vi "DaNIDemoVIveryveryfinal.vi"() -> ()   [LabVIEW 2016]
uses:
  <vilib>/userdefined/High Color/nirio_resource_hc.ctl
  <vilib>/imath/engines/lvmath2/RunTimeEngine/Managers/WorkSpace/UID Generator.vi
  <vilib>/imath/engines/lvmath2/RunTimeEngine/RunTimeType/NIMS_RunTimeType_From StrictType (excl LVString).vi
  <instcachedir>/0/NIMS_RunTimeType_From StrictType (excl LVString)_BBF44FB49F834B71AF7A14CCEDF8BECD.lvgen/NIMS_RunTimeType_From StrictType (excl LVString)_BBF44FB49F834B71AF7A14CCEDF8BECD_000.vi
  <vilib>/imath/engines/lvmath2/RunTimeEngine/LocalVariableDefStatement/MC_LocalVariableDefStatement_Display.vi
  <vilib>/imath/engines/lvmath2/RunTimeEngine/Managers/SymbolTable/Clear UID.vi
  <vilib>/imath/engines/lvmath2/RunTimeEngine/NodeEndStatement/NIMS_NodeEndStatement_Output.vi
  <instcachedir>/0/NIMS_NodeEndStatement_Output_53EC0D466D134D7ABD903AC30B43404B.lvgen/NIMS_NodeEndStatement_Output_53EC0D466D134D7ABD903AC30B43404B_001.vi
  <vilib>/imath/engines/lvmath2/RunTimeEngine/ErrorHandling/NIMS_Finalize Error.vi
  <vilib>/imath/engines/lvmath2/RunTimeEngine/Managers/SymbolTable/NIMS_WorkSpace.lvlib
panel:
  out "x .or. y?":bool
  out "wddot":dbl
  out "vddot":dbl
  in  "Stop Button":bool
  in  "Mode Select":T1(ring)=enum."DaNI Simulation"
  in  "IP Adress":T2="rio://169.254.0.1/RIO0"
  in  "dt (ms)":u32=65
  out "Rad/s Left":dbl
  out "Rad/s Right":dbl
  in  "Left _PID":cluster{"Kp":dbl, "Ti":dbl, "Td":dbl}={"Kp"=0.035, "Ti"=1.25, "Td"=0.0001}
  in  "Right_PID":cluster{"Kp":dbl, "Ti":dbl, "Td":dbl}={"Kp"=0.035, "Ti"=1.5, "Td"=0.0001}
  out "s1 and s2":cluster{"ve":dbl, "we":dbl}(graph)
  out "thetad":dbl
  out "yd":dbl
  out "xd":dbl
  out "w_L":dbl
  out "w_R":dbl
  out "wd":dbl
  out "vd":dbl
  in  "k":cluster{" k0":dbl, "k1":dbl, "k2":dbl}={" k0"=2.0, "k1"=4.0, "k2"=1.1}
  in  "file path (use dialog)":path
  out "error in v and w":cluster{"ve":dbl, "we":dbl}(graph)
  out "error in x y theta":cluster{"xe":dbl, "ye":dbl, "thetae":dbl}(graph)
  out "desired and controlled w":cluster{dbl, "xr+1":dbl}(graph)
  out "desired and controlled v":cluster{dbl, "xr+1":dbl}(graph)
  out "desired and controlled theta":cluster{dbl, "xr+1":dbl}(graph)
  out "desired and controlled trajectory":cluster{dbl[], dbl[]}[](graph)
  out "desired y and controlled y":cluster{dbl, "yr+1":dbl}(graph)
  out "desired x and controlled x":cluster{dbl, "xr+1":dbl}(graph)
  in  "P and Q":cluster{"P1":dbl, "P2":dbl, "Q1":dbl, "Q2":dbl}={"P1"=0.2, "P2"=0.2, "Q1"=0.4, "Q2"=0.4}
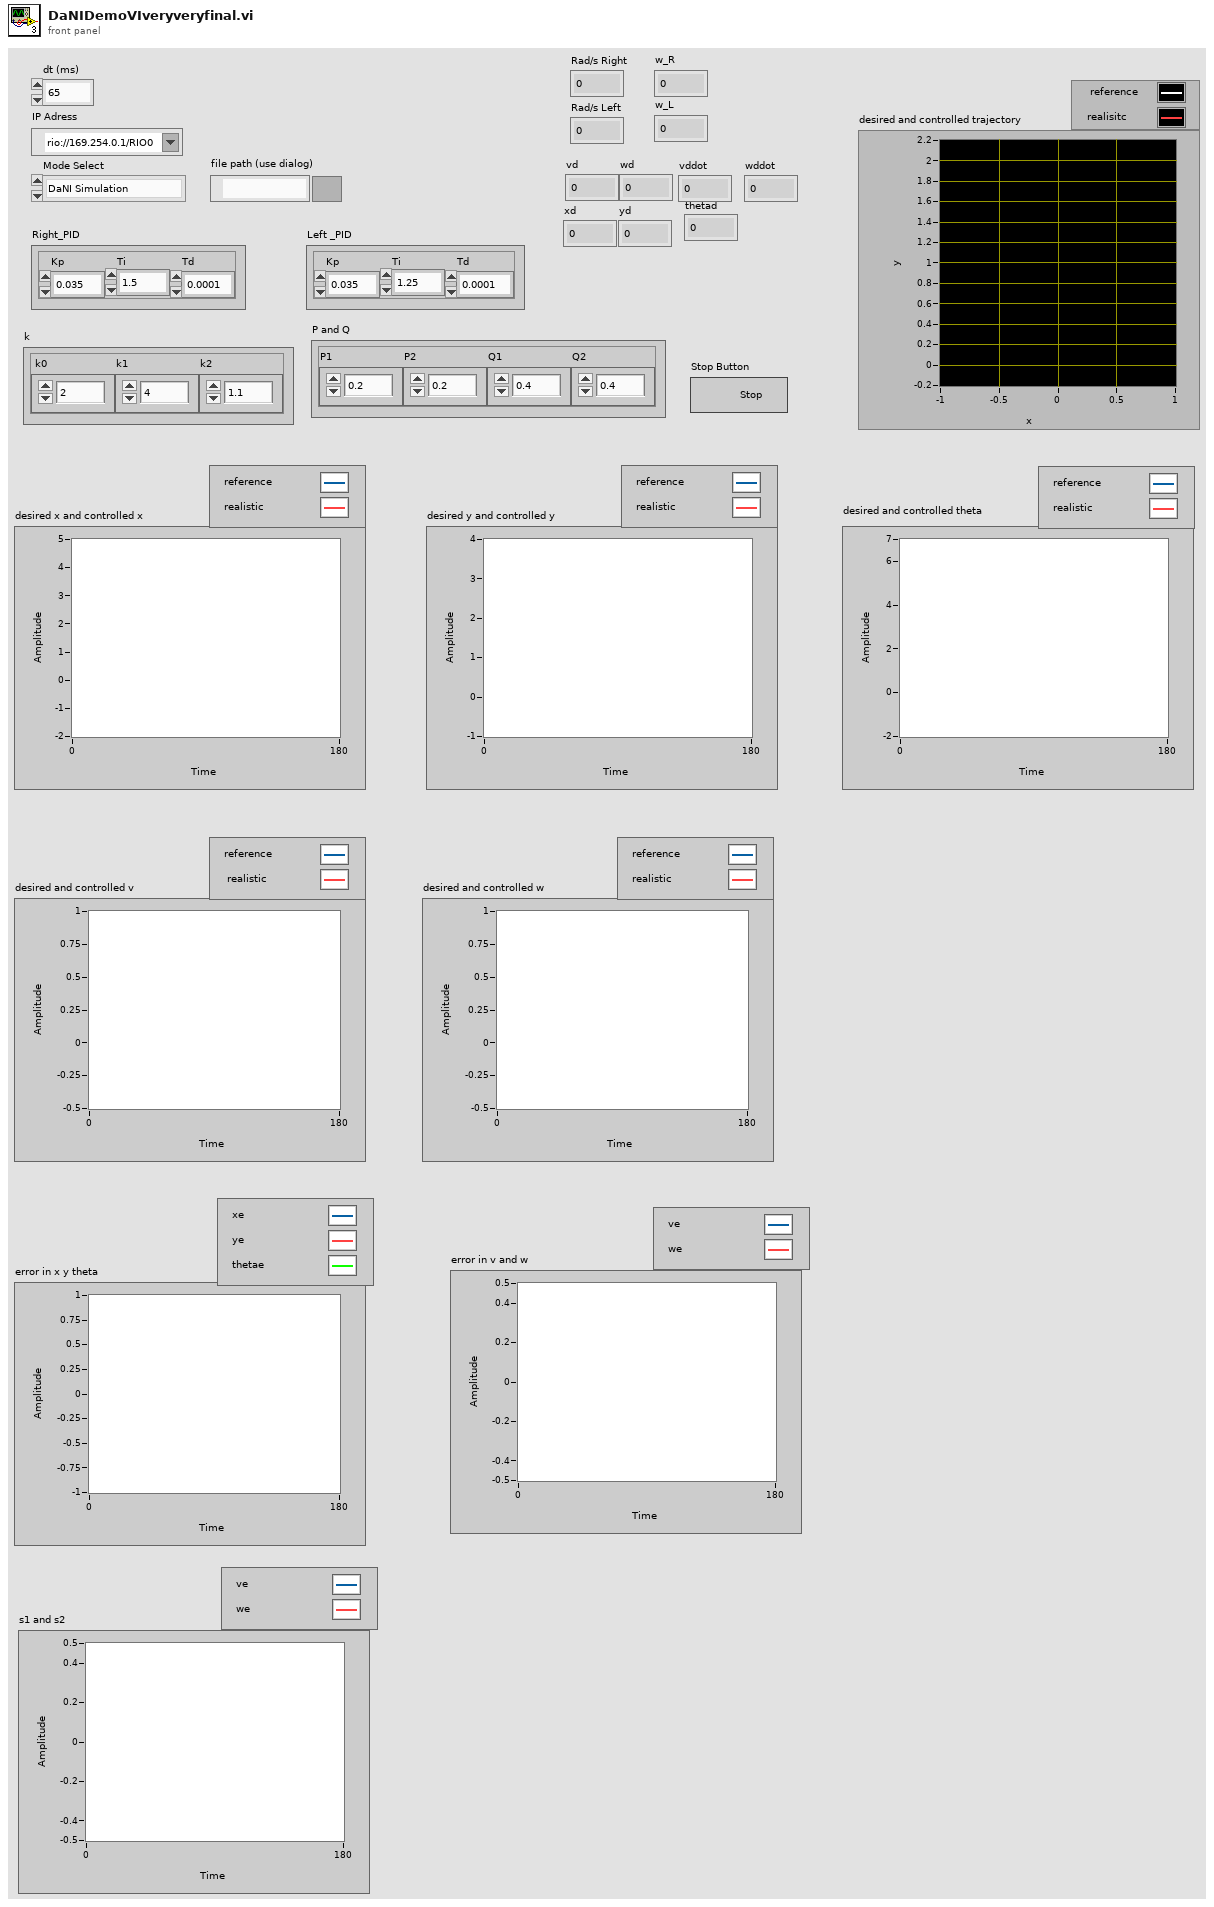
[diagram p1: front panel]
types:
  T1 = enum16{"DaNI DC Motor Sim", "DaNI Simulation", "DaNI Robot"}
  T2 = typedef "nirio_resource_hc.ctl" = tag
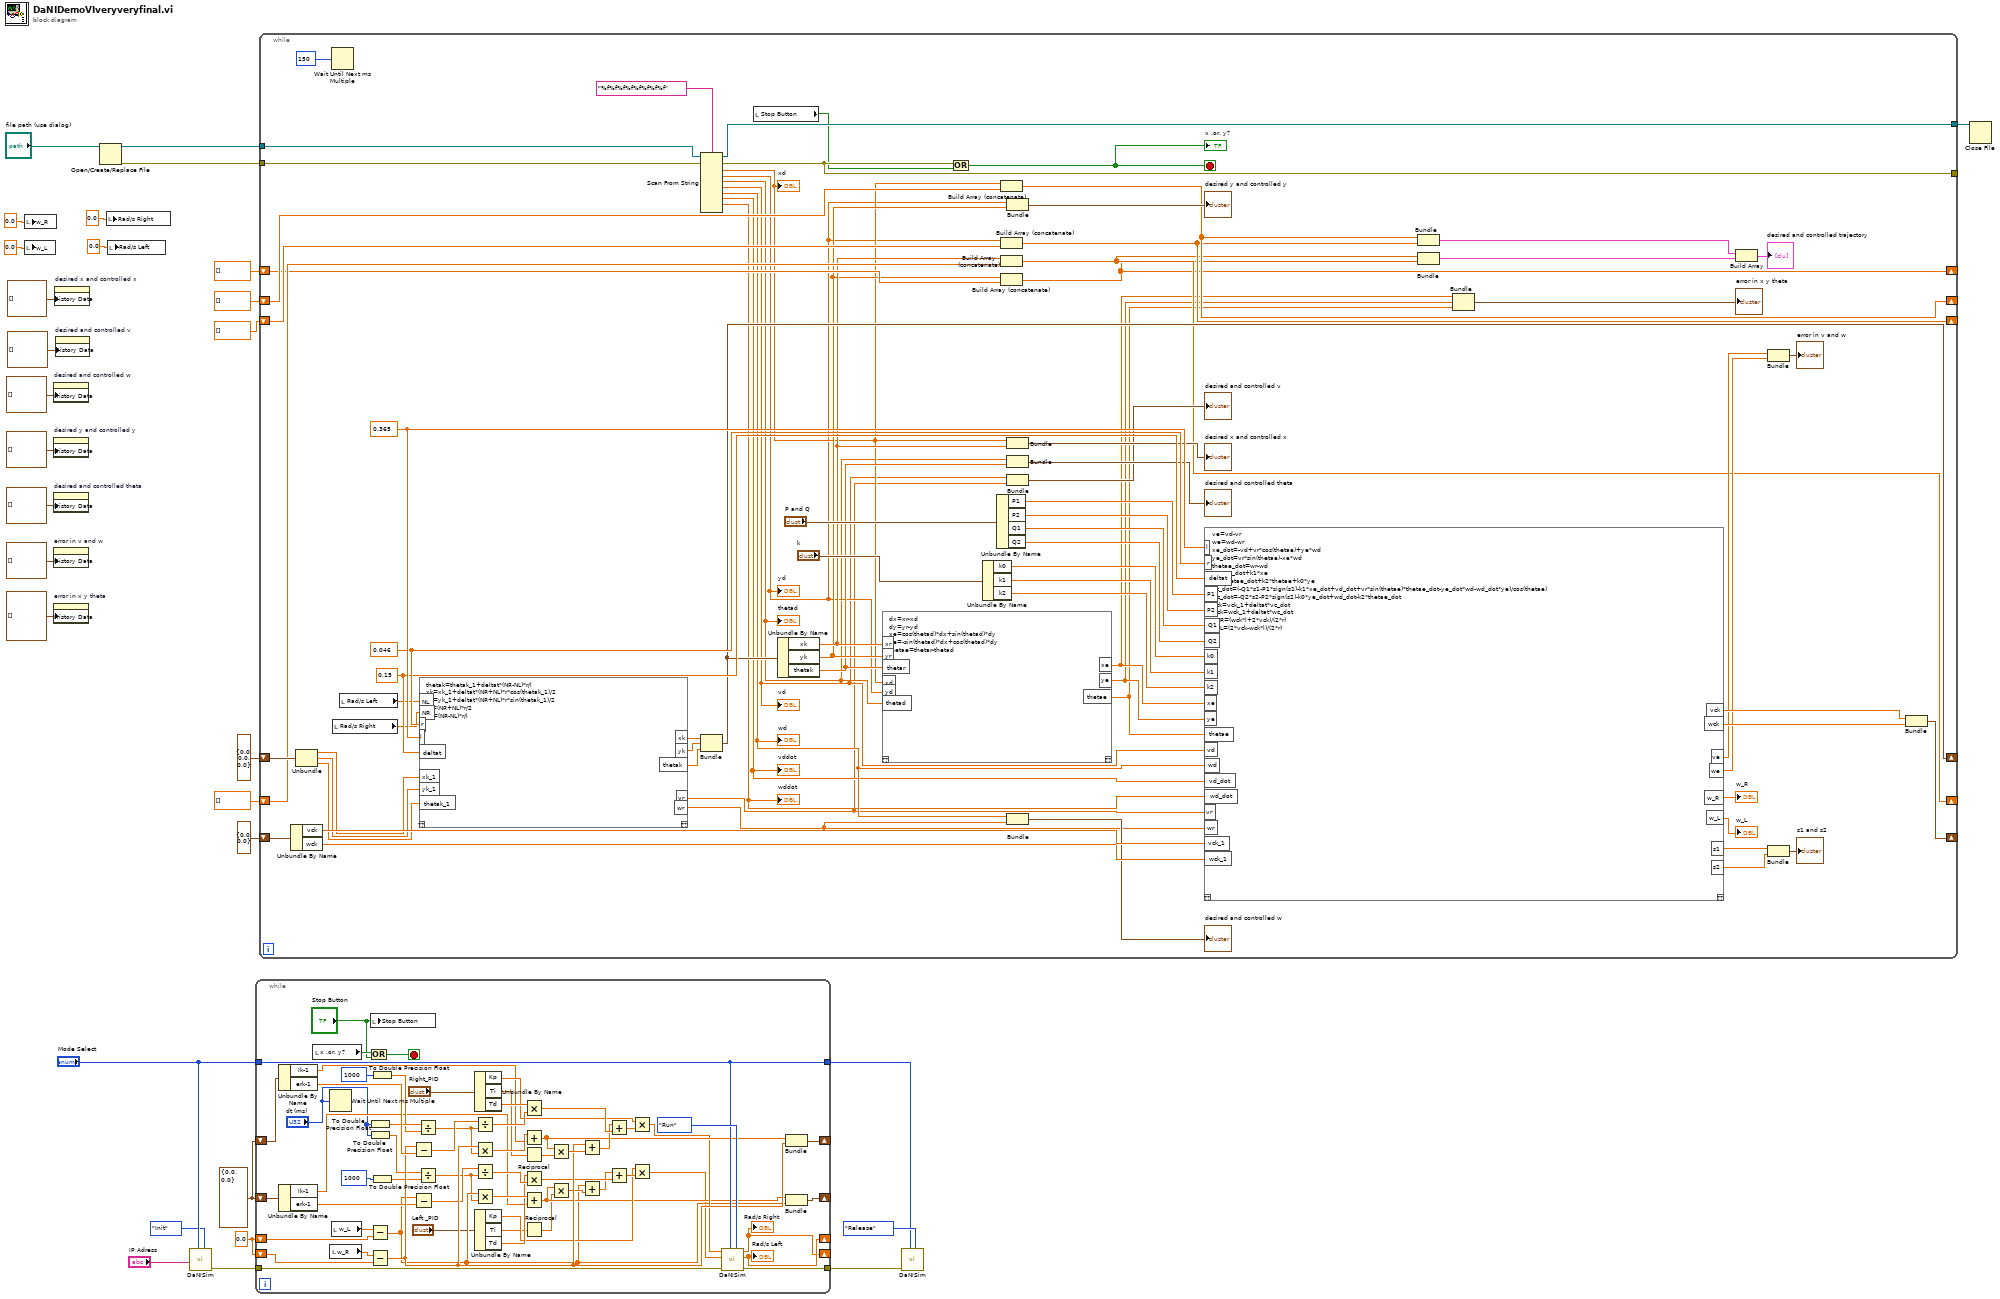
[diagram p0: block diagram]
diagram:
  w9 = 0.0 ("OmegaR")
  w13 = cluster{"Ik-1":dbl, "erk-1":dbl} {"Ik-1"=0.0, "erk-1"=0.0} ("tk-1")
  n1 = local write "w_R"(0.0 ("w_R")) -> ()
  n2 = local write "w_L"(0.0 ("w_L")) -> ()
  n3 = property on="desired and controlled w" class="WFChart (strict)"("History Data"=cluster{dbl, "xr+1":dbl}[] []) -> ()  [unwired: 2 in, 2 out]
  n4 = property on="desired y and controlled y" class="WFChart (strict)"("History Data"=cluster{dbl, "yr+1":dbl}[] []) -> ()  [unwired: 2 in, 2 out]
  n5 = property on="desired and controlled theta" class="WFChart (strict)"("History Data"=cluster{dbl, "xr+1":dbl}[] []) -> ()  [unwired: 2 in, 2 out]
  n6 = property on="error in v and w" class="WFChart (strict)"("History Data"=cluster{"ve":dbl, "we":dbl}[] []) -> ()  [unwired: 2 in, 2 out]
  n7 = property on="error in x y theta" class="WFChart (strict)"("History Data"=cluster{"xe":dbl, "ye":dbl, "thetae":dbl}[] []) -> ()  [unwired: 2 in, 2 out]
  n8 = property on="desired x and controlled x" class="WFChart (strict)"("History Data"=cluster{dbl, "xr+1":dbl}[] []) -> ()  [unwired: 2 in, 2 out]
  n9 = property on="desired and controlled v" class="WFChart (strict)"("History Data"=cluster{dbl, "xr+1":dbl}[] []) -> ()  [unwired: 2 in, 2 out]
  n10 = Open/Create/Replace File(file path (use dialog)="file path (use dialog)") -> (refnum out=w29:refnum<file>, error out=w28:errorcluster)  [unwired: 5 in, 1 out]
  n11 = local write "Rad/s Right"(0.0 ("Rad/s Left")) -> ()
  n12 = local write "Rad/s Left"(0.0 ("Rad/s Right")) -> ()
  n13 = call "DaNISim.vi"("Action"=enum16{"Init", "Run", "Release"}."Init", "Mode Select"="Mode Select", "IP Adress"="IP Adress") -> ("error out"=w5:errorcluster)  [unwired: 5 in, 3 out]
  n14 = while {
    tunnel: w5 -> [w90]
    tunnel: "Mode Select" -> [w85]
    tunnel: [w89] -> w11
    tunnel: [w85] -> w10
    shift-right: [w41] -> _
    shift-left: w13 -> [w40]
    shift-right: [w61] -> _
    shift-left: w13 -> [w62]
    shift-right: [w87] -> _
    shift-left: w9 -> [w65]
    shift-right: [w88] -> _
    shift-left: w9 -> [w37]
    stop <- w31 stop-if-true
    n15 = Unbundle By Name(w62) -> ("Ik-1"=w75:dbl, "erk-1"=w74:dbl)
    n16 = Unbundle By Name(w40) -> ("Ik-1"=w50:dbl, "erk-1"=w49:dbl)
    n17 = local read "x .or. y?"() -> (w33:bool)
    n18 = Wait Until Next ms Multiple(millisecond multiple="dt (ms)") -> ()  [unwired: 1 out]
    n19 = local read "w_R"() -> (w64:dbl)
    n20 = local read "w_L"() -> (w38:dbl)
    n21 = Or(x=w33, y="Stop Button") -> (x .or. y?=w31:bool)
    n22 = To Double Precision Float(number="dt (ms)") -> (double precision float=w70:dbl)
    n23 = To Double Precision Float(number="dt (ms)") -> (double precision float=w45:dbl)
    n24 = Subtract(x=w38, y=w37) -> (x-y=w47:dbl)
    n25 = Subtract(x=w64, y=w65) -> (x-y=w72:dbl)
    n26 = local write "Stop Button"("Stop Button") -> ()
    n27 = To Double Precision Float(number=1000) -> (double precision float=w69:dbl)
    n28 = To Double Precision Float(number=1000) -> (double precision float=w44:dbl)
    n29 = Subtract(x=w72, y=w74) -> (x-y=w83:dbl)
    n30 = Subtract(x=w47, y=w49) -> (x-y=w58:dbl)
    n31 = Divide(x=w70, y=w69) -> (x/y=w66:dbl)
    n32 = Divide(x=w45, y=w44) -> (x/y=w43:dbl)
    n33 = Unbundle By Name("Right_PID") -> ("Kp"=w76:dbl, "Ti"=w68:dbl, "Td"=w77:dbl)
    n34 = Divide(x=w83, y=w66) -> (x/y=w84:dbl)
    n35 = Multiply(x=w72, y=w66) -> (x*y=w79:dbl)
    n36 = Divide(x=w58, y=w43) -> (x/y=w59:dbl)
    n37 = Multiply(x=w47, y=w43) -> (x*y=w54:dbl)
    n38 = Unbundle By Name("Left _PID") -> ("Kp"=w51:dbl, "Ti"=w35:dbl, "Td"=w52:dbl)
    n39 = Multiply(x=w77, y=w84) -> (x*y=w82:dbl)
    n40 = Add(x=w79, y=w75) -> (x+y=w73:dbl)
    n41 = Reciprocal(x=w68) -> (1/x=w67:dbl)
    n42 = Multiply(x=w52, y=w59) -> (x*y=w57:dbl)
    n43 = Add(x=w54, y=w50) -> (x+y=w48:dbl)
    n44 = Reciprocal(x=w35) -> (1/x=w34:dbl)
    n45 = Multiply(x=w73, y=w67) -> (x*y=w78:dbl)
    n46 = Multiply(x=w48, y=w34) -> (x*y=w53:dbl)
    n47 = Add(x=w72, y=w78) -> (x+y=w81:dbl)
    n48 = Add(x=w47, y=w53) -> (x+y=w56:dbl)
    n49 = Add(x=w81, y=w82) -> (x+y=w80:dbl)
    n50 = Add(x=w56, y=w57) -> (x+y=w55:dbl)
    n51 = Multiply(x=w76, y=w80) -> (x*y=w60:dbl)
    n52 = Multiply(x=w51, y=w55) -> (x*y=w36:dbl)
    n53 = call "DaNISim.vi"("Action"=enum16{"Init", "Run", "Release"}."Run", "Mode Select"=w85, "error in (no error)"=w90, "Ul"=w36, "Ur"=w60) -> ("error out"=w89:errorcluster, "OmegaL"=w88:dbl, "OmegaR"=w87:dbl)  [unwired: 3 in, 1 out]
    "Rad/s Left" <- w88
    "Rad/s Right" <- w87
    n54 = Bundle(w73, w72) -> (w61:cluster{dbl, dbl})  [unwired: 1 in]
    n55 = Bundle(w48, w47) -> (w41:cluster{dbl, dbl})  [unwired: 1 in]
  }
  n56 = while {
    shift-right: [w122] -> _
    shift-left: cluster{"xr+1":dbl, "yr+1":dbl, "thetar+1":dbl} {"xr+1"=0.0, "yr+1"=0.0, "thetar+1"=0.0} ("real x y theta (k+1)") -> [w135]
    tunnel: w29 -> [w165]
    shift-right: [w140] -> _
    shift-left: cluster{"vck":dbl, "wck":dbl} {"vck"=0.0, "wck"=0.0} ("vck wck") -> [w156]
    tunnel: w28 -> [w163]
    tunnel: [w160] -> w27
    tunnel: [w159] -> _
    shift-right: [w113] -> _
    shift-left: dbl[] [] -> [w112]
    shift-right: [w110] -> _
    shift-left: dbl[] [] -> [w111]
    shift-right: [w108] -> _
    shift-left: dbl[] [] -> [w109]
    shift-right: [w107] -> _
    shift-left: dbl[] [] -> [w106]
    stop <- w162 stop-if-true
    w131 = 0.365 ("l")
    w130 = 0.046 ("r")
    w129 = 0.15 ("deltat")
    n57 = Unbundle By Name(w156) -> ("vck"=w148:dbl, "wck"=w147:dbl)
    n58 = Unbundle(w135) -> ("xr+1"=w134:dbl, "yr+1"=w133:dbl, "thetar+1"=w132:dbl)
    n59 = Wait Until Next ms Multiple(millisecond multiple=u32 150 ("Embedded PC dt (ms)")) -> ()  [unwired: 1 out]
    n60 = local read "Rad/s Right"() -> (w128:dbl)
    n61 = local read "Rad/s Left"() -> (w127:dbl)
    n62 = mathscript code="thetak=thetak_1+deltat*(NR-NL)*r/l\nxk=xk_1+deltat*(NR+NL)*r*cos(thetak_1)/2\nyk=yk_1+deltat*(NR+NL)*r*sin(thetak_1)/2\nvr=(NR+NL)*r/2\nwr=(NR-NL)*r/l"("NL"=w127, "NR"=w128, "r"=w130, "l"=w131, "deltat"=w129, "xk_1"=w134, "yk_1"=w133, "thetak_1"=w132) -> ("xk"=w138:dbl, "yk"=w137:dbl, "thetak"=w136:dbl, "vr"=w92:dbl, "wr"=w91:dbl)  [unwired: 1 in, 1 out]
    n63 = Scan From String ("Scan From File")("%f%f%f%f%f%f%f%f", w165, w163) -> (w160:refnum<file>, w159:errorcluster, output 1=w99:dbl, output 2=w98:dbl, output 3=w97:dbl, output 4=w96:dbl, output 5=w95:dbl, output 6=w93:dbl, output 7=w94:dbl)  [unwired: 9 in]
    "vd" <- w96
    "wd" <- w95
    "xd" <- w99
    "yd" <- w98
    "thetad" <- w97
    "vddot" <- w93
    "wddot" <- w94
    n64 = Bundle("xk"=w138, "yk"=w137, "thetak"=w136) -> (w122:cluster{"xk":dbl, "yk":dbl, "thetak":dbl})  [unwired: 1 in]
    n65 = local read "Stop Button"() -> (w115:bool)
    n66 = Unbundle By Name(w122) -> ("xk"=w102:dbl, "yk"=w101:dbl, "thetak"=w100:dbl)
    n67 = mathscript code="dx=xr-xd\ndy=yr-yd\nxe=cos(thetad)*dx+sin(thetad)*dy\nye=-sin(thetad)*dx+cos(thetad)*dy\nthetae=thetar-thetad"("xr"=w102, "yr"=w101, "thetar"=w100, "xd"=w99, "yd"=w98, "thetad"=w97) -> ("xe"=w105:dbl, "ye"=w104:dbl, "thetae"=w103:dbl)  [unwired: 1 in, 1 out]
    n68 = Or(x=w159, y=w115) -> (x .or. y?=w162:bool)
    "x .or. y?" <- w162
    n69 = Unbundle By Name("k") -> ("k0"=w151:dbl, "k1"=w150:dbl, "k2"=w149:dbl)
    n70 = Unbundle By Name("P and Q") -> ("P1"=w155:dbl, "P2"=w154:dbl, "Q1"=w153:dbl, "Q2"=w152:dbl)
    n71 = Build Array (concatenate)(w99, w112) -> (w113:dbl[])
    n72 = Build Array (concatenate)(w98, w111) -> (w110:dbl[])
    n73 = Build Array (concatenate)(w102, w109) -> (w108:dbl[])
    n74 = Build Array (concatenate)(w101, w106) -> (w107:dbl[])
    n75 = Bundle("yd"=w98, "yk"=w101) -> (→"desired y and controlled y":cluster{"yd":dbl, "yk":dbl})  [unwired: 1 in]
    n76 = Bundle("xd"=w99, "xk"=w102) -> (→"desired x and controlled x":cluster{"xd":dbl, "xk":dbl})  [unwired: 1 in]
    n77 = Bundle("thetad"=w97, "thetak"=w100) -> (→"desired and controlled theta":cluster{"thetad":dbl, "thetak":dbl})  [unwired: 1 in]
    n78 = Bundle("vd"=w96, "vr"=w92) -> (→"desired and controlled v":cluster{"vd":dbl, "vr":dbl})  [unwired: 1 in]
    n79 = Bundle("wd"=w95, "wr"=w91) -> (→"desired and controlled w":cluster{"wd":dbl, "wr":dbl})  [unwired: 1 in]
    n80 = mathscript code="ve=vd-vr\nwe=wd-wr\nxe_dot=-vd+vr*cos(thetae)+ye*wd\nye_dot=vr*sin(thetae)-xe*wd\nthetae_dot=wr-wd\ns1=xe_dot+k1*xe\ns2=thetae_dot+k2*thetae+k0*ye\nvc_dot=(-Q1*s1-P1*sign(s1)-k1*xe_dot+vd_dot+vr*sin(thetae)*thetae_dot-ye_dot*wd-wd_dot*ye)/cos(thetae)\nwc_dot=-Q2*s2-P2*sign(s2)-k0*ye_dot+wd_dot-k2*thetae_dot\nvck=vck_1+deltat*vc_dot\nwck=wck_1+deltat*wc_dot\nw_R=(wck*l+2*vck)/(2*r)\nw_L=(2*vck-wck*l)/(2*r)"("l"=w131, "r"=w130, "P1"=w155, "P2"=w154, "Q1"=w153, "Q2"=w152, "k0"=w151, "k1"=w150, "k2"=w149, "xe"=w105, "ye"=w104, "thetae"=w103, "vd"=w96, "wd"=w95, "vd_dot"=w93, "wd_dot"=w94, "vr"=w92, "wr"=w91, "vck_1"=w148, "wck_1"=w147, "deltat"=w129) -> ("w_R"=→"w_R":dbl, "w_L"=→"w_L":dbl, "vck"=w145:dbl, "wck"=w146:dbl, "we"=w141:dbl, "ve"=w142:dbl, "s1"=w118:dbl, "s2"=w117:dbl)  [unwired: 1 in, 1 out]
    n81 = Bundle(w113, w110) -> (w161:cluster{dbl[], dbl[]})  [unwired: 1 in]
    n82 = Bundle(w108, w107) -> (w121:cluster{dbl[], dbl[]})  [unwired: 1 in]
    n83 = Bundle("xe"=w105, "ye"=w104, "thetae"=w103) -> (→"error in x y theta":cluster{"xe":dbl, "ye":dbl, "thetae":dbl})  [unwired: 1 in]
    n84 = Build Array(w161, w121) -> (→"desired and controlled trajectory":cluster{dbl[], dbl[]}[])
    n85 = Bundle("ve"=w142, "we"=w141) -> (→"error in v and w":cluster{"ve":dbl, "we":dbl})  [unwired: 1 in]
    n86 = Bundle("s1"=w118, "s2"=w117) -> (→"s1 and s2":cluster{"s1":dbl, "s2":dbl})  [unwired: 1 in]
    n87 = Bundle("vck"=w145, "wck"=w146) -> (w140:cluster{"vck":dbl, "wck":dbl})  [unwired: 1 in]
  }
  n88 = call "DaNISim.vi"("Action"=enum16{"Init", "Run", "Release"}."Release", "Mode Select"=w10, "error in (no error)"=w11) -> ()  [unwired: 5 in, 4 out]
  n89 = Close File(refnum=w27) -> ()  [unwired: 1 in, 2 out]
